vi "Riccati_DARE_StructDoubling.vi"(8 "R":T1, 9 "Q":T1, 10 "B":T1, 11 "A":T1) -> (0 "error out":errorcluster, 1 "Error":bool, 2 "Iterations":i32, 3 "Answer":T1)   [LabVIEW 2019, in "Trajectory_Library.lvlib"]
doc: "Solves the discrete alegebraic Riccati equation.\n\nThis uses an iterative method to arrive at the solution. Run time is not deterministic and this routine should not be used during run-time, only during initialization.\n \nInput:\n - A -- System matrix.\n - B -- nput matrix.\n - Q -- State cost matrix.\n - R -- Input cost matrix.\n\nOutputs:\n Answer -- Solution of DARE.\n iterations -- Number of iterations\n error -- If TRUE, an error occured"
uses:
  Trajectory_Library.lvlib
  <vilib>/Analysis/Matrix/Datatypes/RealMatrix.ctl
  <vilib>/Analysis/baseanly.llb/Real A x B.vi
  <vilib>/Analysis/baseanly.llb/Real Inverse Matrix.vi
  <vilib>/Analysis/7linalg.llb/Create Special Matrix.vi
  <vilib>/Analysis/7linalg.llb/Create Special Real Matrix.vi
  <vilib>/Analysis/Matrix/Numeric/Add/Add - RM,RM.vi
  <vilib>/Analysis/Matrix/Numeric/Subtract/Subtract - RM,RM.vi
  <vilib>/Analysis/Matrix/Numeric/Multiply/Multiply - RM,R.vi
  <vilib>/Analysis/NI_AALBase.lvlib
  <vilib>/Analysis/Matrix/NI_Matrix.lvlib
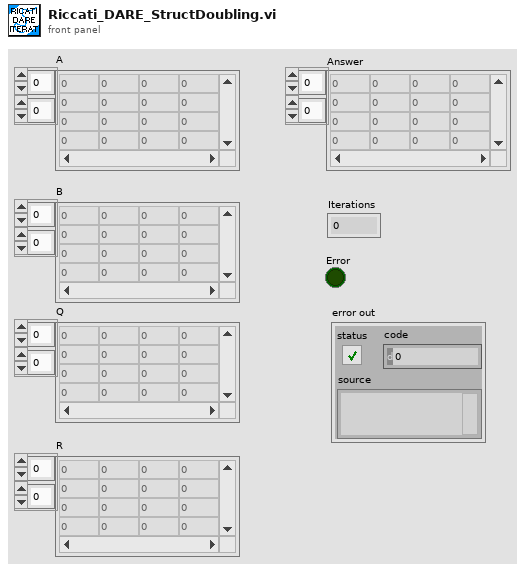
[diagram p1: front panel]
types:
  T1 = typedef "NI_Matrix.lvlib/RealMatrix.ctl" = dbl[][]
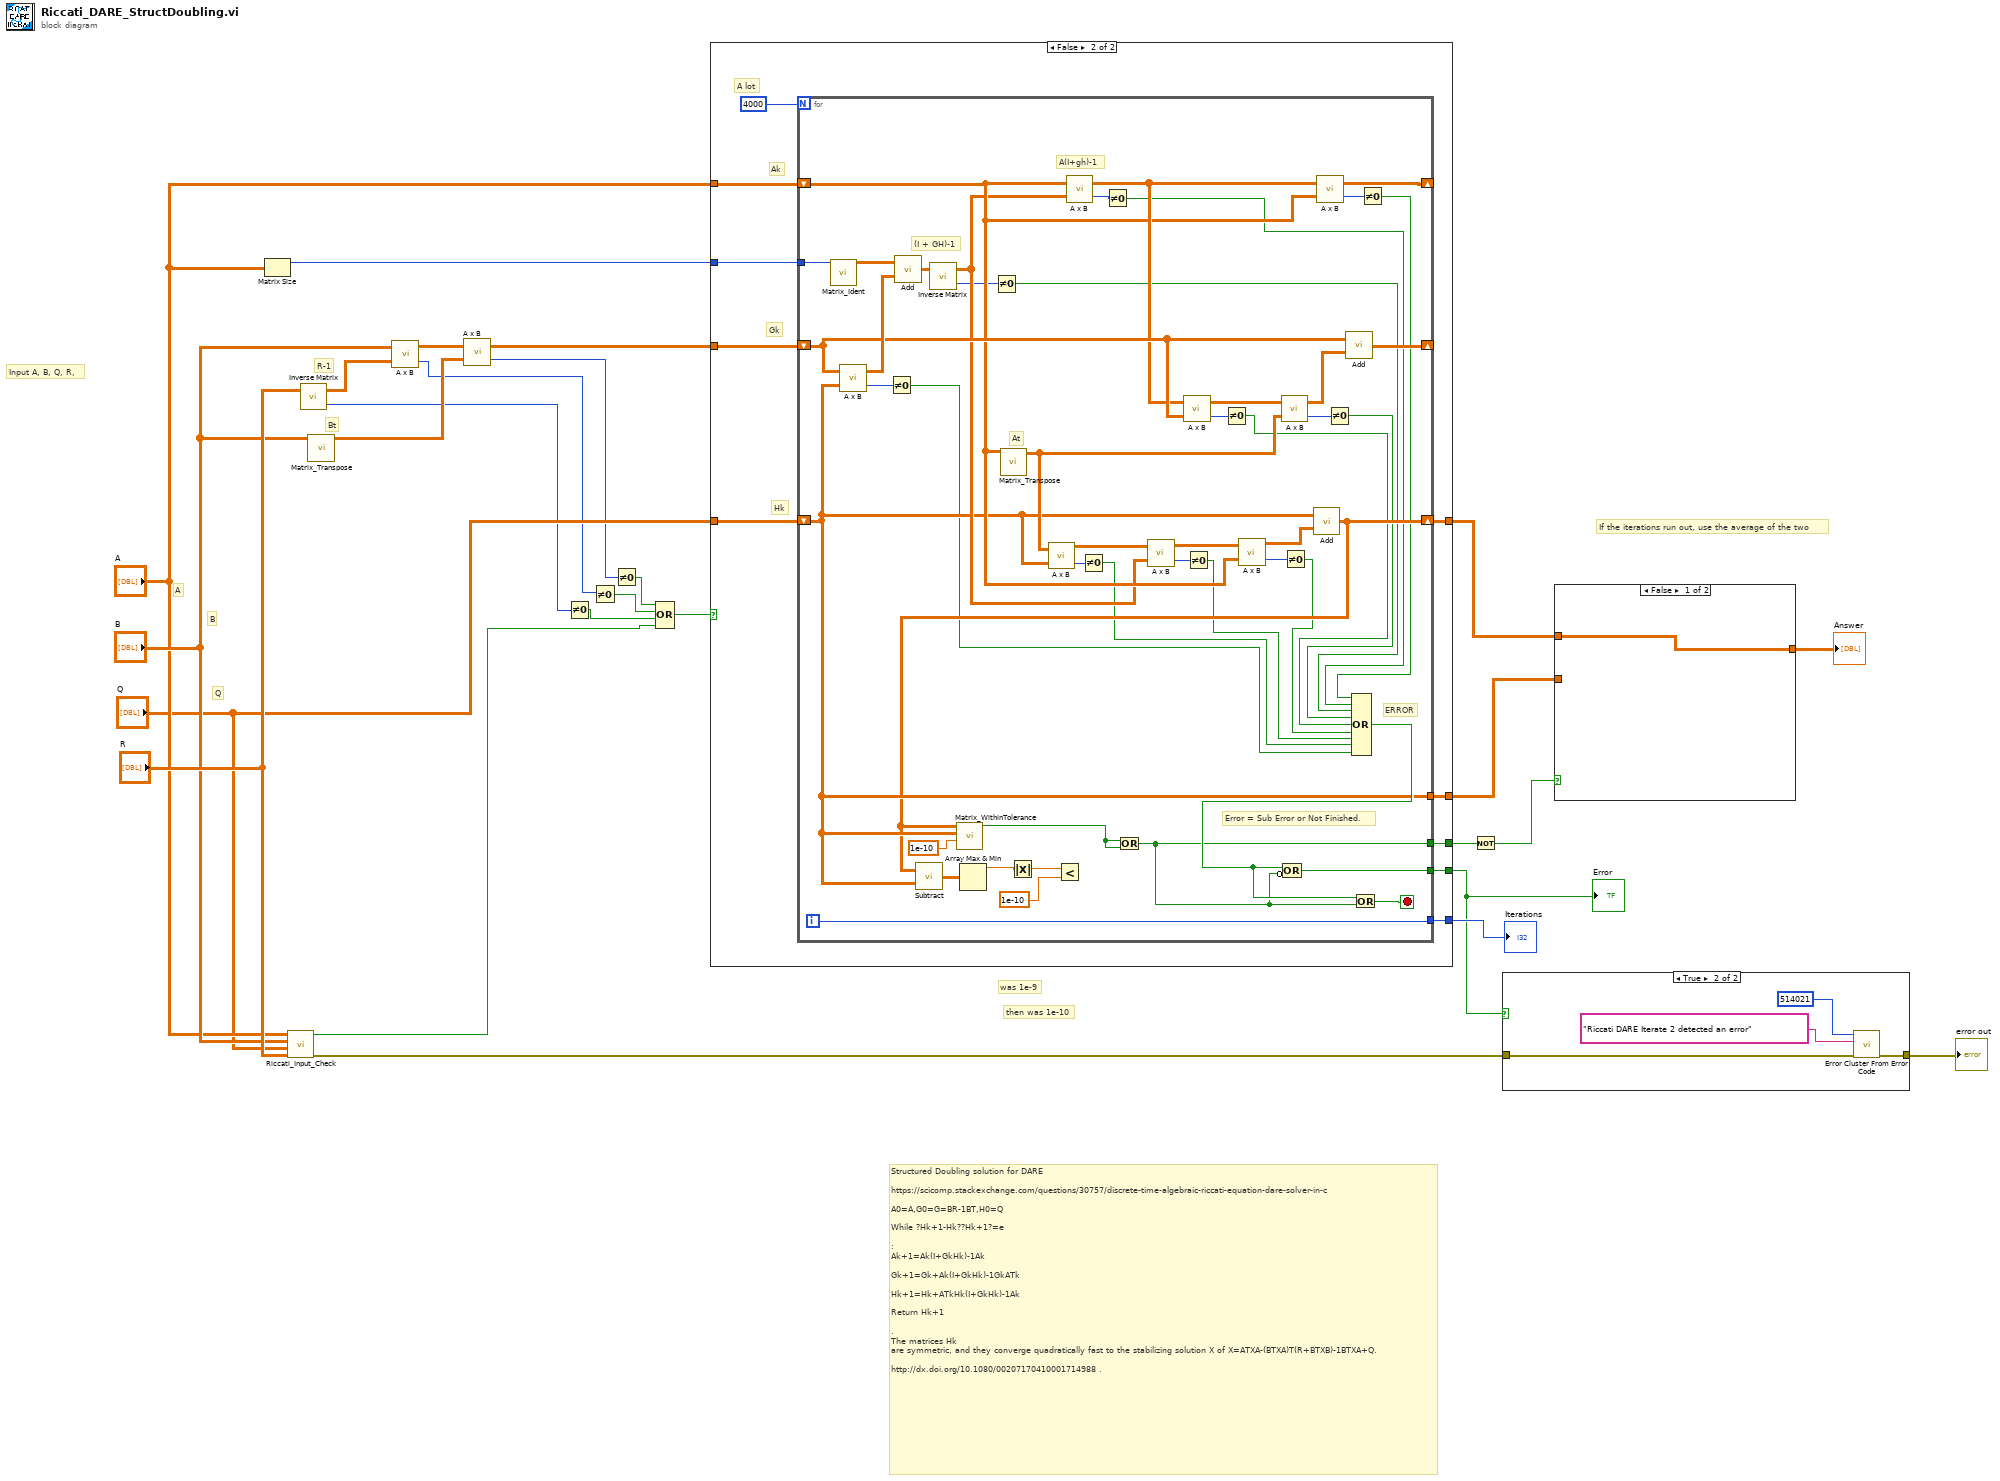
[diagram p0: block diagram]
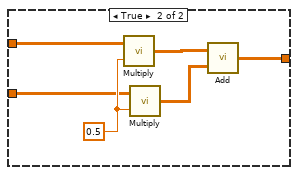
[diagram p2: hidden frame]
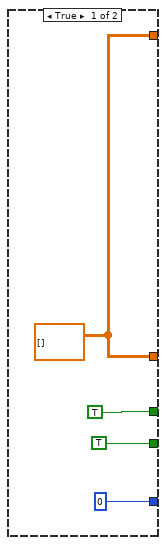
[diagram p4: hidden frame]
diagram:
  # "Structured Doubling solution for DARE\n\nhttps://scicomp.stackexchange.com/questions/30757/discrete-time-algebraic-riccati-equation-dare-solver-in-c\n\nA0=A,G0=G=BR-1BT,H0=Q\n\nWhile ?Hk+1-Hk??Hk+1?=e\n\n:\nAk+1=Ak(I+GkHk)-1Ak\n\nGk+1=Gk+Ak(I+GkHk)-1GkATk\n\nHk+1=Hk+ATkHk(I+GkHk)-1Ak\n\nReturn Hk+1\n\n.\nThe matrices Hk\nare symmetric, and they converge quadratically fast to the stabilizing solution X of X=ATXA-(BTXA)T(R+BTXB)-1BTXA+Q.\n\nhttp://dx.doi.org/10.1080/00207170410001714988 ."
  # "If the iterations run out, use the average of the two"
  # "then was 1e-10"
  # "was 1e-9"
  # "B"
  # "R-1"
  # "Bt"
  # "Q"
  # "A"
  # "Input A, B, Q, R,"
  n1 = Matrix Size(0:"A") -> (1:w15:i32)  [unwired: 1 out]
  n2 = call "Riccati_Input_Check.vi"("R"="R", "Q"="Q", "B"="B", "A"="A") -> ("error out"=w22:errorcluster, "Error"=w5:bool)  [unwired: 6 in]
  n3 = call-poly <vilib>:"Inverse Matrix.vi"("Input Matrix"="R") -> ("error"=w1:i32, "Inverse Matrix"=w11:T1)  [unwired: 1 in]
  n4 = call "Matrix_Transpose.vi"("input matrix"="B") -> ("output matrix"=w9:T1)  [unwired: 10 in]
  n5 = call-poly <vilib>:"A x B.vi"("B"=w11, "A"="B") -> ("error"=w2:i32, "A x B"=w10:T1)
  n6 = call-poly <vilib>:"A x B.vi"("B"=w9, "A"=w10) -> ("error"=w3:i32, "A x B"=w7:T1)
  n7 = Not Equal To 0?(x=w1) -> (x != 0?=w6:bool)
  n8 = Not Equal To 0?(x=w2) -> (x != 0?=w25:bool)
  n9 = Not Equal To 0?(x=w3) -> (x != 0?=w13:bool)
  n10 = Compound Arithmetic op=OR(w13, w25, w6, w5) -> (w12:bool)
  n11 = case shown="False" w12 {
    tunnel: [w27 w31] -> w18
    tunnel: [0 w39] -> w26
    tunnel: [TRUE w38] -> w23
    tunnel: [TRUE ("WithinTolerance") w37] -> w20
    tunnel: [w27 w36] -> w16
    tunnel: w15 -> [_ w35]
    tunnel: "A" -> [_ w34]
    tunnel: w7 -> [_ w33]
    tunnel: "Q" -> [_ w32]
    frame True {
      w27 = T1 [] ("Q")
    }
    frame False {
      # "Hk"
      # "Gk"
      # "Ak"
      # "A lot"
      n12 = for {
        N: 4000 -> [_]
        tunnel: [w87] -> w39
        tunnel: [w81] -> w38
        tunnel: [w59] -> w37
        tunnel: [w61] -> w36
        tunnel: w35 -> [w78]
        shift-right: [w76] -> _
        shift-left: w34 -> [w64]
        shift-right: [w71] -> _
        shift-left: w33 -> [w69]
        shift-right: [w60] -> w31
        shift-left: w32 -> [w61]
        i -> [w87]
        stop <- w82 stop-if-true
        # "At"
        # "A(I+gh)-1"
        # "(I + GH)-1"
        # "Error = Sub Error or Not Finished."
        # "ERROR"
        n13 = call "Matrix_Ident.vi"("Size"=w78) -> ("output matrix"=w75:T1)  [unwired: 9 in, 1 out]
        n14 = call-poly <vilib>:"A x B.vi"("B"=w61, "A"=w69) -> ("error"=w55:i32, "A x B"=w74:T1)
        n15 = Not Equal To 0?(x=w55) -> (x != 0?=w41:bool)
        n16 = call-poly <vilib>:"Add.vi"("Real Matrix B"=w74, "Real Matrix A"=w75) -> ("A + B"=w73:T1)
        n17 = call-poly <vilib>:"Inverse Matrix.vi"("Input Matrix"=w73) -> ("error"=w56:i32, "Inverse Matrix"=w62:T1)  [unwired: 1 in]
        n18 = Not Equal To 0?(x=w56) -> (x != 0?=w50:bool)
        n19 = call "Matrix_Transpose.vi"("input matrix"=w64) -> ("output matrix"=w68:T1)  [unwired: 10 in]
        n20 = call-poly <vilib>:"A x B.vi"("B"=w61, "A"=w68) -> ("error"=w54:i32, "A x B"=w66:T1)
        n21 = call-poly <vilib>:"A x B.vi"("B"=w62, "A"=w64) -> ("error"=w58:i32, "A x B"=w67:T1)
        n22 = Not Equal To 0?(x=w54) -> (x != 0?=w42:bool)
        n23 = Not Equal To 0?(x=w58) -> (x != 0?=w51:bool)
        n24 = call-poly <vilib>:"A x B.vi"("B"=w62, "A"=w66) -> ("error"=w45:i32, "A x B"=w65:T1)
        n25 = call-poly <vilib>:"A x B.vi"("B"=w69, "A"=w67) -> ("error"=w53:i32, "A x B"=w72:T1)
        n26 = Not Equal To 0?(x=w45) -> (x != 0?=w43:bool)
        n27 = Not Equal To 0?(x=w53) -> (x != 0?=w47:bool)
        n28 = call-poly <vilib>:"A x B.vi"("B"=w64, "A"=w65) -> ("error"=w46:i32, "A x B"=w63:T1)
        n29 = call-poly <vilib>:"A x B.vi"("B"=w68, "A"=w72) -> ("error"=w49:i32, "A x B"=w70:T1)
        n30 = Not Equal To 0?(x=w46) -> (x != 0?=w44:bool)
        n31 = call-poly <vilib>:"Add.vi"("Real Matrix B"=w63, "Real Matrix A"=w61) -> ("A + B"=w60:T1)
        n32 = call-poly <vilib>:"Subtract.vi"("Real Matrix B"=w61, "Real Matrix A"=w60) -> ("A - B"=w86:T1)
        n33 = call "Matrix_WithinTolerance.vi"("Tolerance"=1e-10, "Matrix B"=w61, "Matrix A"=w60) -> ("WithinTolerance"=w77:bool)  [unwired: 7 in, 1 out]
        n34 = Array Max & Min(array=w86) -> (max value=w85:dbl)  [unwired: 3 out]
        n35 = Absolute Value(x=w85) -> (abs(x)=w84:dbl)
        n36 = Less?(x=w84, y=1e-10) -> ()  [unwired: 1 out]
        n37 = Or(x=w77, y=w77) -> (x .or. y?=w59:bool)
        n38 = call-poly <vilib>:"A x B.vi"("B"=w64, "A"=w67) -> ("error"=w57:i32, "A x B"=w76:T1)
        n39 = Not Equal To 0?(x=w49) -> (x != 0?=w48:bool)
        n40 = call-poly <vilib>:"Add.vi"("Real Matrix B"=w70, "Real Matrix A"=w69) -> ("A + B"=w71:T1)
        n41 = Not Equal To 0?(x=w57) -> (x != 0?=w52:bool)
        n42 = Compound Arithmetic op=OR(w52, w51, w50, w48, w47, w44, w43, w42, w41) -> (w80:bool)
        n43 = Compound Arithmetic op=OR(w80, invert w59) -> (w81:bool)
        n44 = Or(x=w80, y=w59) -> (x .or. y?=w82:bool)
      }
    }
  }
  "Iterations" <- w26
  "Error" <- w23
  n45 = Not(x=w20) -> (.not. x?=w19:bool)
  n46 = case shown="True" w23 {
    tunnel: w22 -> [w88 w89]
    tunnel: [w88 w91] -> w21
    frame False {
    }
    frame True {
      n47 = call <vilib>:"Error Cluster From Error Code.vi"("error in (no error)"=w89, "error message (\"\")"="Riccati DARE Iterate 2 detected an error" ("error message (\"\")"), "error code (0)"=514021) -> ("error out"=w91:errorcluster)  [unwired: 6 in]
    }
  }
  "error out" <- w21
  n48 = case shown="False" w19 {
    tunnel: w18 -> [w93 w98]
    tunnel: [w93 w94] -> w17
    tunnel: w16 -> [_ w97]
    frame False {
    }
    frame True {
      w99 = 0.5
      n49 = call-poly <vilib>:"Multiply.vi"("Real Scalar c"=w99, "Real Matrix A"=w98) -> ("A * c"=w96:T1)
      n50 = call-poly <vilib>:"Multiply.vi"("Real Scalar c"=w99, "Real Matrix A"=w97) -> ("A * c"=w95:T1)
      n51 = call-poly <vilib>:"Add.vi"("Real Matrix B"=w95, "Real Matrix A"=w96) -> ("A + B"=w94:T1)
    }
  }
  "Answer" <- w17
